vi "MIDI - Producer.vi"(8 "error in (no error)":errorcluster, 10 "queue in":refnum<queue>, 11 "Refnum in":refnum<k20>) -> (0 "error out":errorcluster)   [LabVIEW 2014]
uses:
  Controls/Application Data.vi
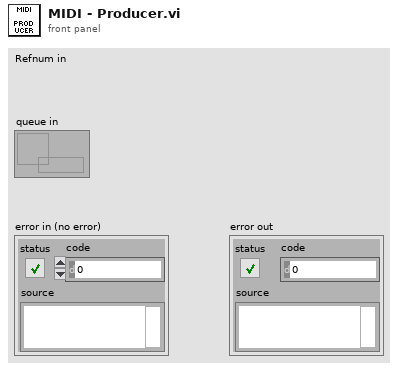
[diagram p1: front panel]
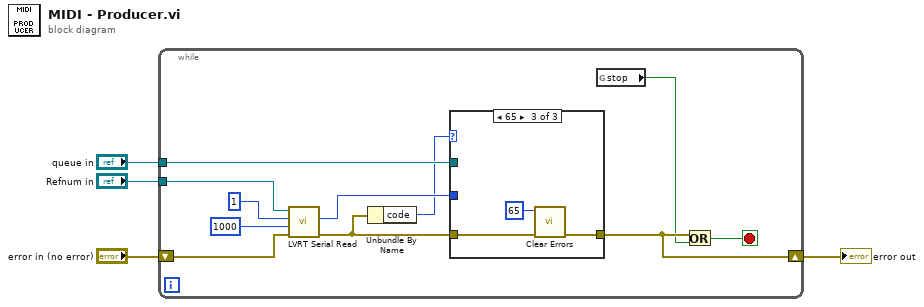
[diagram p0: block diagram]
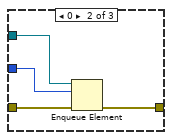
[diagram p3: hidden frame]
diagram:
  n1 = while {
    tunnel: "Refnum in" -> [w13]
    tunnel: "queue in" -> [w11]
    shift-right: [w6] -> w4
    shift-left: "error in (no error)" -> [w8]
    stop <- w7 stop-if-true
    n2 = call "LVRT Serial Read.vi"("error in (no error)"=w8, "Timeout (ms) (-1: no timeout)"=1000 ("Timeout (ms)\n(-1: None)"), "Bytes to Read"=u32 1 ("Character Count"), "FPGA Main Ref"=w13) -> ("error out"=w10:errorcluster, "Read: Char"=w12:u8)  [unwired: 6 out]
    n3 = Unbundle By Name(w10) -> ("code"=w9:i32)
    n4 = case shown="65" w9 {
      tunnel: w10 -> [w16 w19 w23]
      tunnel: w11 -> [_ w20 _]
      tunnel: [w16 w18 w22] -> w6
      tunnel: w12 -> [_ w17 _]
      frame 1, Default {
      }
      frame 0 {
        n5 = Enqueue Element(queue=w20, element=w17, error in (no error)=w19) -> (error out=w18:errorcluster)  [unwired: 1 in, 2 out]
      }
      frame 65 {
        n6 = call <vilib>:"Clear Errors.vi"("error in (no error)"=w23, "specific error code to clear (0: all)"=65) -> ("error out"=w22:errorcluster)  [unwired: 4 in, 1 out]
      }
    }
    n7 = global read "Application Data.vi" "stop"() -> (w5:bool)
    n8 = Or(x=w6, y=w5) -> (x .or. y?=w7:bool)
  }
  "error out" <- w4
